vi "Control-Indicador de alarmas de temperatura.vi"() -> ()   [LabVIEW 2019]
panel:
  out "Boolean 3":bool
  out "Boolean 2":bool
  out "Boolean":bool
  in  "Knob":dbl(knob) scale=0.0..100.0
  out "Temperatura en C°":dbl(slide) scale=0.0..100.0
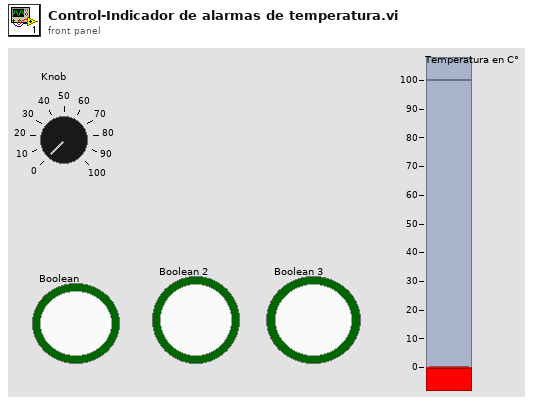
[diagram p1: front panel]
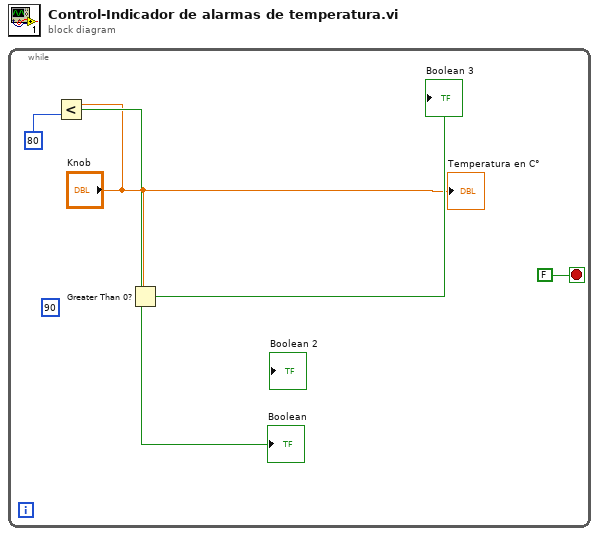
[diagram p0: block diagram]
diagram:
  n1 = while {
    stop <- FALSE stop-if-true
    (unwired) 90
    n2 = Less?(x="Knob", y=80) -> (x < y?=→"Boolean":bool)
    n3 = Greater Than 0?(x="Knob") -> (x > 0?=→"Boolean 3":bool)
    "Temperatura en C°" <- "Knob"
  }
